vi "Odour_sequences.vi"() -> ()   [LabVIEW 2016]
panel:
  in  "Sequences":T1(array[cluster]) {"Reward condition" items=["None", "Both / middle", "Left", "Right", "No-go"]}
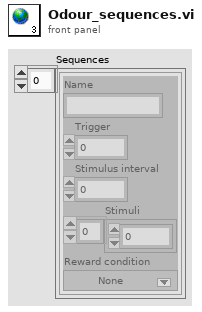
[diagram p1: front panel]
types:
  T1 = cluster{"Name":string, "Trigger":u16, "Stimulus interval":dbl, "Stimuli":i32[], "Reward condition":u16}[]
diagram:
